vi "发送.vi"(1 "数据（32bit）":string, 2 "命令(16bit)":string, 3 "目标IP":string="192.168.0.2") -> (0 "错误输出":errorcluster)   [LabVIEW 2014]
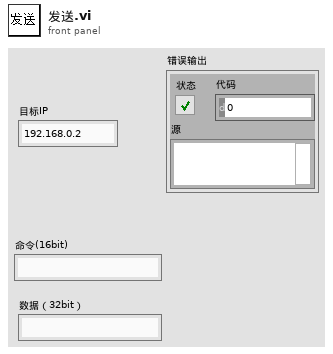
[diagram p1: front panel]
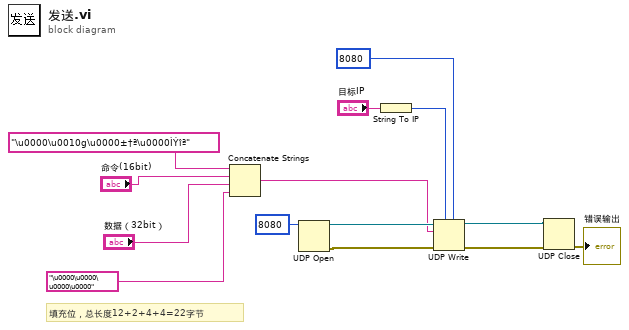
[diagram p0: block diagram]
diagram:
  # "填充位，总长度12+2+4+4=22字节"
  n1 = Concatenate Strings("\u0000\u0010g\u0000±†ª\u0000ÌÝîª" ("字符串"), "命令(16bit)", "数据（32bit）", "\u0000\u0000\u0000\u0000" ("字符串")) -> (w3:string)
  n2 = UDP Open(11:u16 8080 ("端口")) -> (port=w13:refnum<k16>, 0:w12:errorcluster)  [unwired: 4 in, 1 out]
  n3 = String To IP(1:"目标IP") -> (0:w11:u32)
  n4 = UDP Write(address=w11, port or service name=u16 8080 ("端口或服务名称"), connection ID=w13, data in=w3, 8:w12) -> (error out=w7:errorcluster, 3:w8:refnum<k16>)  [unwired: 1 in]
  n5 = UDP Close(connection ID=w8, 8:w7) -> (error out=→"错误输出":errorcluster)  [unwired: 1 out]
